vi "Execute Command.vi"(8 "error in (no error)":errorcluster, 10 "Slide Panel in":refnum<class "Slide Panel Off Screen.lvclass">, 11 "User Interface References":T1={"This VI"=refnum, "User Interace Plugin"=refnum, "UI Picture Container References"={"Header Image"=refnum, "Footer Image"=refnum}, "Sliding Menu XControl"=refnum, "Menu Container"=refnum, "UI Configuration Information"={"Space Between Buttons"=3, "Number of Buttons to Show"=6, "Header Image"=path "Images/Blue Background.bmp", "Footer Image"=path "Images/Blue Background.bmp"}, "Header Text"=refnum}) -> (0 "error out":errorcluster, 1 "Stop?":bool, 2 "Slide Panel out":refnum<class "Slide Panel Off Screen.lvclass">, 3 "User Interface References Out":T1={"This VI"=refnum, "User Interace Plugin"=refnum, "UI Picture Container References"={"Header Image"=refnum, "Footer Image"=refnum}, "Sliding Menu XControl"=refnum, "Menu Container"=refnum, "UI Configuration Information"={"Space Between Buttons"=3, "Number of Buttons to Show"=6, "Header Image"=path "Images/Blue Background.bmp", "Footer Image"=path "Images/Blue Background.bmp"}, "Header Text"=refnum})   [LabVIEW 2011, in "Slide Panel Off Screen.lvclass"]
uses:
  Slide Panel Off Screen.lvclass
  Main Type Definitions/User Interface Type Definitions.ctl
  Main Type Definitions/UI Picture Containers.ctl
  Sliding Menu/Sliding Menu Library/Sliding Menu xControl/Sliding Menu XControl.xctl
  UI Control Definitions/UI Configuration Information.ctl
  <vilib>/Utility/miscctls.llb/LVPositionTypeDef.ctl
  <vilib>/Utility/miscctls.llb/LVRectTypeDef.ctl
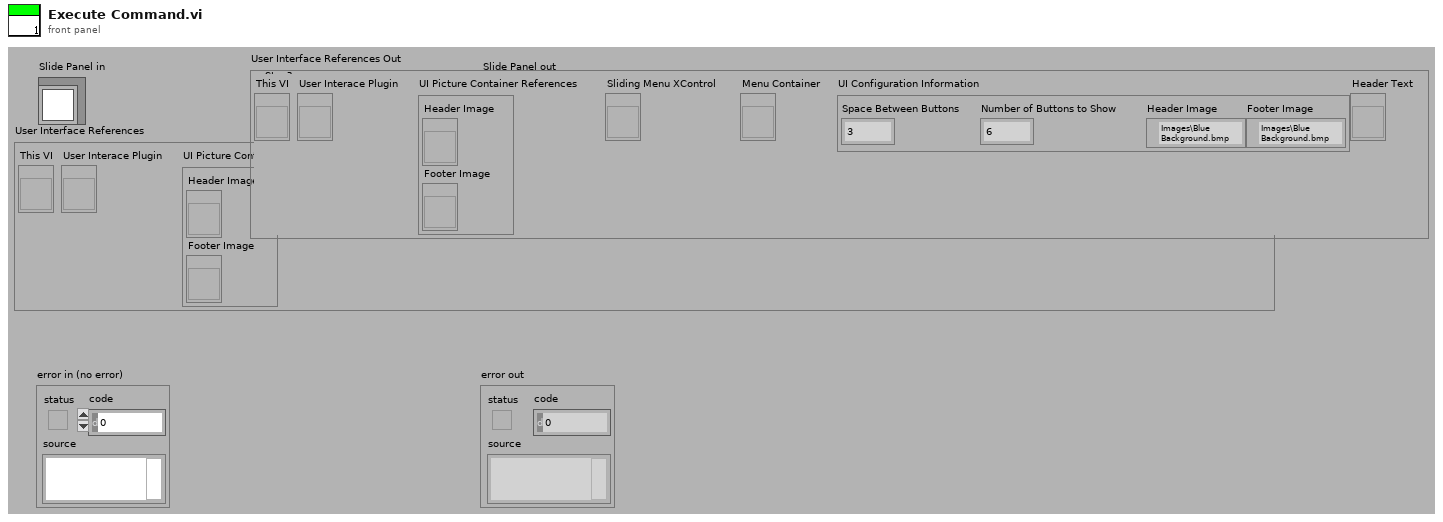
[diagram p1: front panel]
types:
  T1 = typedef "User Interface Type Definitions.ctl" = cluster{"This VI":refnum<vi>, "User Interace Plugin":refnum<vi>, "UI Picture Container References":T2, "Sliding Menu XControl":refnum<vi>, "Menu Container":refnum<vi>, "UI Configuration Information":T3, "Header Text":refnum<vi>}
  T2 = typedef "UI Picture Containers.ctl" = cluster{"Header Image":refnum<vi>, "Footer Image":refnum<vi>}
  T3 = typedef "UI Configuration Information.ctl" = cluster{"Space Between Buttons":i32, "Number of Buttons to Show":i32, "Header Image":path, "Footer Image":path}
  T4 = typedef "LVPositionTypeDef.ctl" = cluster{"Left":i32, "Top":i32}
  T5 = typedef "LVRectTypeDef.ctl" = cluster{"Left":i16, "Top":i16, "Right":i16, "Bottom":i16}
  T6 = typedef "LVBoundsTypeDef.ctl" = cluster{"Width":u32, "Height":u32}
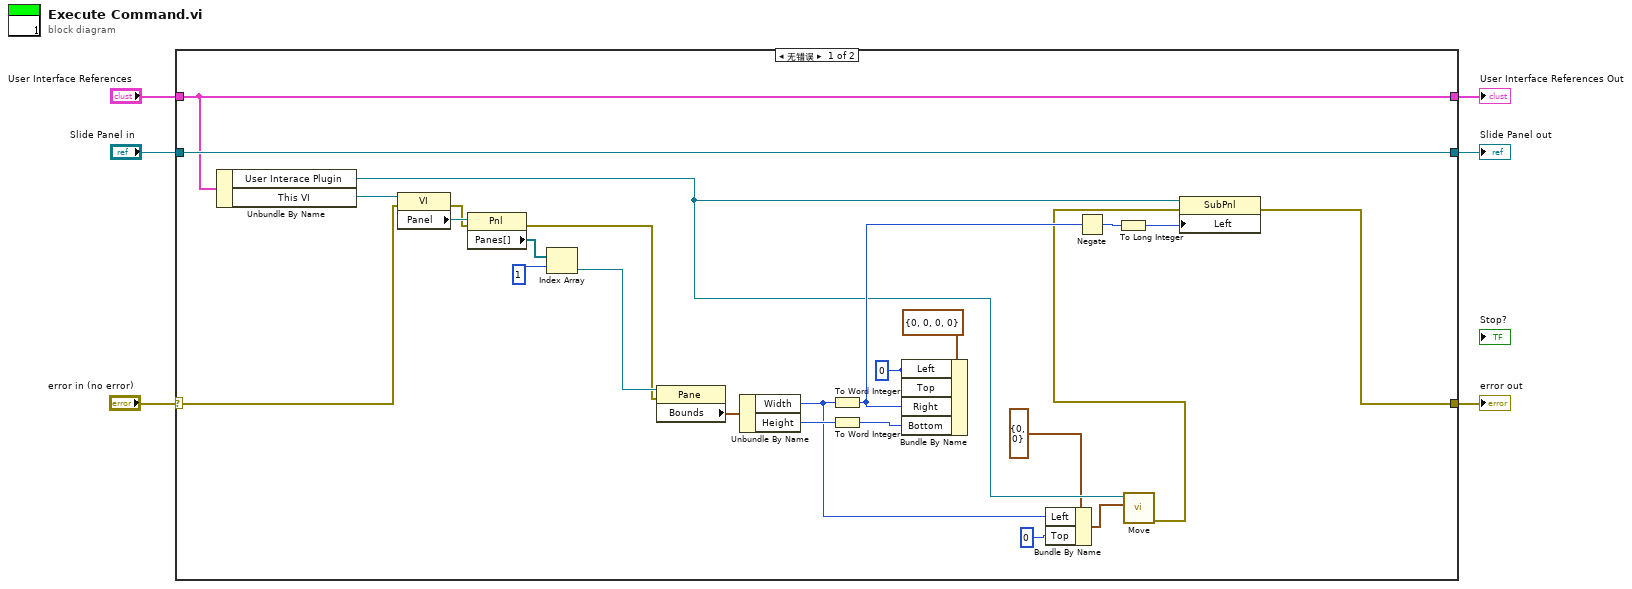
[diagram p0: block diagram]
diagram:
  n1 = case shown="无错误" "error in (no error)" {
    selector: "error in (no error)" -> [w17 w32]
    tunnel: [w30 w34] -> w4
    tunnel: "User Interface References" -> [w30 w34]
    tunnel: [w31 w33] -> w2
    tunnel: "Slide Panel in" -> [w31 w33]
    tunnel: [w13 w32] -> w1
    frame No Error {
      w18 = i16 0 ("Right")
      n2 = Unbundle By Name(w30) -> ("User Interace Plugin"=w12:refnum<vi>, "This VI"=w29:refnum<vi>)
      n3 = property class="VI"(reference=w29, error in=w17) -> (error out=w23:errorcluster, "Panel"=w28:refnum<vi>)  [unwired: 1 out]
      n4 = property class="Pnl"(reference=w28, error in=w23) -> (error out=w24:errorcluster, "Panes[]"=w27:refnum<vi>[])  [unwired: 1 out]
      n5 = Index Array(array=w27, index=1) -> (element=w25:refnum<vi>)
      n6 = property class="Pane"(reference=w25, error in=w24) -> ("Bounds"=w21:T6)  [unwired: 2 out]
      n7 = Unbundle By Name(w21) -> ("Width"=w9:u32, "Height"=w20:u32)
      n8 = To Word Integer(number=w9) -> (16bit integer=w16:i16)
      n9 = To Word Integer(number=w20) -> (16bit integer=w19:i16)
      n10 = Bundle By Name(cluster=T5 {"Left"=0, "Top"=0, "Right"=0, "Bottom"=0} ("Frame Bounds"), "Left"=w18, "Top"=w18, "Right"=w16, "Bottom"=w19) -> ()  [unwired: 1 out]
      n11 = Bundle By Name(cluster=T4 {"Left"=0, "Top"=0} ("Desired Position"), "Left"=w9, "Top"=0) -> (w10:T4)
      n12 = Negate(x=w16) -> (-x=w14:i16)
      n13 = To Long Integer(number=w14) -> (32bit integer=w15:i32)
      n14 = call "Move.vi"("Desired Position"=w10, "Obj Ref"=w12) -> ("error out"=w7:errorcluster)  [unwired: 7 in, 2 out]
      n15 = property class="SubPnl"(reference=w12, error in=w7, "Left"=w15) -> (error out=w13:errorcluster)  [unwired: 1 out]
    }
    frame Error {
    }
  }
  "error out" <- w1
  "Slide Panel out" <- w2
  "User Interface References Out" <- w4
